vi "Build Multi Line SQL CMD1.vi"(7 "DB Type":T1(ring), 11 "Data Array":string[][](array[string])) -> (3 "String":string)   [LabVIEW 2021]
doc: "INSERT INTO NoteID\n(\nNoteID,Type,Enable,Notes\n)\n VALUES"
uses:
  <userlib>/LabSQL/LabSQL.lvlib
panel:
  # "INSERT INTO NoteID\n(\nNoteID,Type,Enable,Notes\n)\n VALUES"
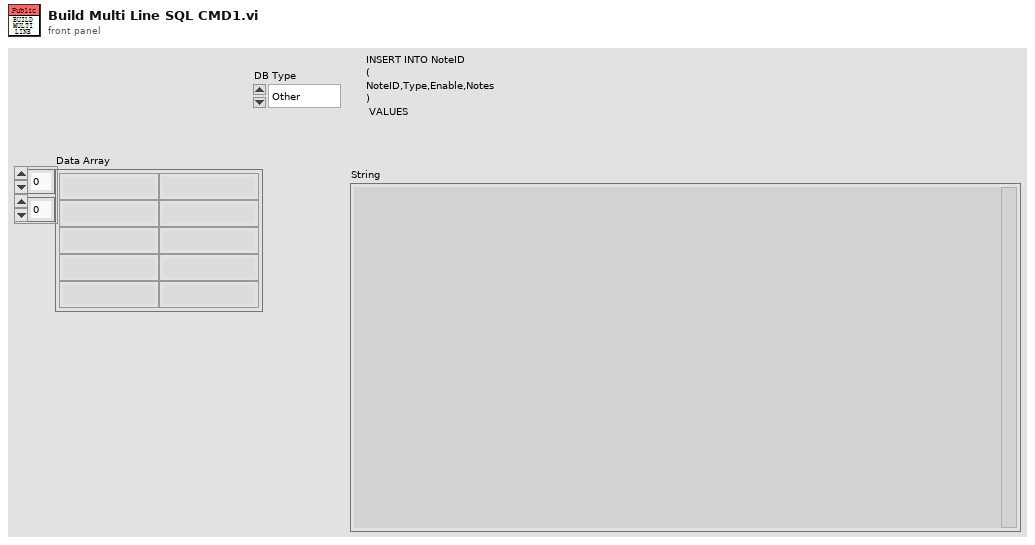
[diagram p1: front panel]
types:
  T1 = enum16{"Other", "SQL2008", "SQLite", "Access", "MySQL"}
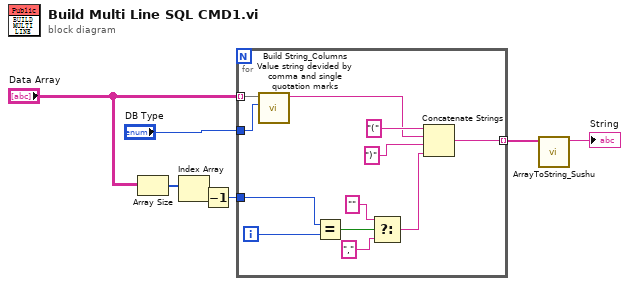
[diagram p0: block diagram]
diagram:
  n1 = Array Size(array="Data Array") -> (size(s)=w4:i32[])
  n2 = Index Array(array=w4) -> (element=w5:i32)  [unwired: 1 in]
  n3 = Decrement(x=w5) -> (x-1=w7:i32)
  n4 = for {
    tunnel: "Data Array" -> [w19] mode=indexing
    tunnel: [w15] -> w2 mode=indexing
    tunnel: "DB Type" -> [w14]
    tunnel: w7 -> [w13]
    i -> [w12]
    n5 = call <userlib>:"Build String_Columns Value string devided by comma and single quotation marks.vi"("DB Type 2"=w14, "ColumnsValueList"=w19) -> ("ColumnsValuesString"=w16:string)  [unwired: 9 in]
    n6 = Equal?(x=w13, y=w12) -> (x = y?=w11:bool)
    n7 = Select(t="", s=w11, f="," ("string")) -> (s? t:f=w9:string)
    n8 = Concatenate Strings("(" ("string"), w16, ")" ("string"), w9) -> (w15:string)
  }
  n9 = call <userlib>:"ArrayToString_Sushu.vi"("Array"=w2) -> ("String"=→"String":string)  [unwired: 10 in]
